vi "Is Cluster.vi"(8 "Error In":errorcluster, 11 "GObject In":refnum<vi>) -> (0 "Error Out":errorcluster, 2 "Cluster?":bool, 3 "GObject Out":refnum<vi>)   [LabVIEW 2017, in "Toolkit.lvlib"]
doc: "Checks if the GObject reference is to a cluster constant on the Block Diagram or a cluster control on the Front Panel."
uses:
  Toolkit.lvlib
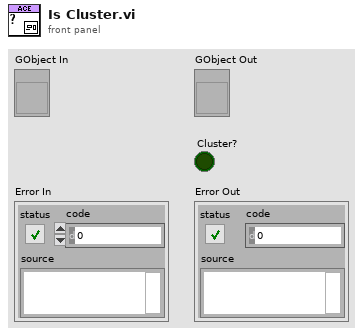
[diagram p1: front panel]
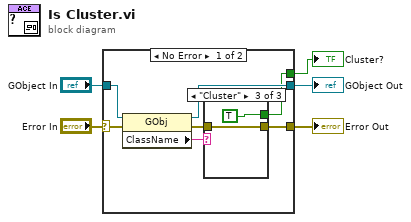
[diagram p0: block diagram]
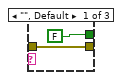
[diagram p2: hidden frame]
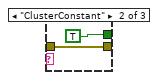
[diagram p3: hidden frame]
diagram:
  n1 = case shown="No Error" "Error In" {
    selector: "Error In" -> [w12 w20]
    tunnel: [w11 w20] -> w4
    tunnel: [w6 _] -> w3
    tunnel: "GObject In" -> [w8 w19]
    tunnel: [w7 w19] -> w1
    frame No Error {
      n2 = property class="GObj"(reference=w8, error in=w12) -> (reference out=w7:refnum<vi>, error out=w9:errorcluster, "ClassName"=w10:string)
      n3 = case shown="\"Cluster\"" w10 {
        tunnel: w9 -> [w14 w15 w17]
        tunnel: [w14 w15 w17] -> w11
        tunnel: [FALSE TRUE TRUE] -> w6
        frame "", Default {
        }
        frame "ClusterConstant" {
        }
        frame "Cluster" {
        }
      }
    }
    frame Error {
    }
  }
  "Error Out" <- w4
  "Cluster?" <- w3
  "GObject Out" <- w1
